vi "Test - Draw Teapot.vi"() -> ()   [LabVIEW 2022 SP3, in "Raster.lvlib"] (continued)
"UV"={"u"=0.0, "v"=0.0}, "Colour"=12517256}, "Vertex 2"={"Position"={"x"=274.62903, "y"=381.50693, "z"=0.99085957}, "UV"={"u"=0.0, "v"=0.0}, "Colour"=12517256}, "Vertex 3"={"Position"={"x"=264.3577, "y"=384.847, "z"=0.9904829}, "UV"={"u"=0.0, "v"=0.0}, "Colour"=12517256}, "Alpha"=0.0, "Alpha Blending Enabled"=FALSE, "Colour"=6654024}, {"Vertex 1"={"Position"={"x"=274.78113, "y"=379.6353, "z"=0.99085855}, "UV"={"u"=0.0, "v"=0.0}, "Colour"=12517256}, "Vertex 2"={"Position"={"x"=274.32074, "y"=376.97778, "z"=0.99086154}, "UV"={"u"=0.0, "v"=0.0}, "Colour"=12517256}, "Vertex 3"={"Position"={"x"=264.01044, "y"=380.14035, "z"=0.99048406}, "UV"={"u"=0.0, "v"=0.0}, "Colour"=12517256}, "Alpha"=0.0, "Alpha Blending Enabled"=FALSE, "Colour"=329219}, {"Vertex 1"={"Position"={"x"=525.67926, "y"=376.97778, "z"=0.99086154}, "UV"={"u"=0.0, "v"=0.0}, "Colour"=12517256}, "Vertex 2"={"Position"={"x"=525.2189, "y"=379.6353, "z"=0.99085855}, "UV"={"u"=0.0, "v"=0.0}, "Colour"=12517256}, "Vertex 3"={"Position"={"x"=535.4709, "y"=382.89456, "z"=0.99048245}, "UV"={"u"=0.0, "v"=0.0}, "Colour"=12517256}, "Alpha"=0.0, "Alpha Blending Enabled"=FALSE, "Colour"=329219}, {"Vertex 1"={"Position"={"x"=525.2189, "y"=379.6353, "z"=0.99085855}, "UV"={"u"=0.0, "v"=0.0}, "Colour"=12517256}, "Vertex 2"={"Position"={"x"=525.371, "y"=381.50693, "z"=0.99085957}, "UV"={"u"=0.0, "v"=0.0}, "Colour"=12517256}, "Vertex 3"={"Position"={"x"=535.6423, "y"=384.847, "z"=0.9904829}, "UV"={"u"=0.0, "v"=0.0}, "Colour"=12517256}, "Alpha"=0.0, "Alpha Blending Enabled"=FALSE, "Colour"=2898719}, {"Vertex 1"={"Position"={"x"=274.62903, "y"=381.50693, "z"=0.99085957}, "UV"={"u"=0.0, "v"=0.0}, "Colour"=12517256}, "Vertex 2"={"Position"={"x"=274.78113, "y"=379.6353, "z"=0.99085855}, "UV"={"u"=0.0, "v"=0.0}, "Colour"=12517256}, "Vertex 3"={"Position"={"x"=264.52908, "y"=382.89456, "z"=0.99048245}, "UV"={"u"=0.0, "v"=0.0}, "Colour"=12517256}, "Alpha"=0.0, "Alpha Blending Enabled"=FALSE, "Colour"=2898719}, {"Vertex 1"={"Position"={"x"=263.60925, "y"=385.99985, "z"=0.99048537}, "UV"={"u"=0.0, "v"=0.0}, "Colour"=12517256}, "Vertex 2"={"Position"={"x"=262.39697, "y"=386.3562, "z"=0.99048924}, "UV"={"u"=0.0, "v"=0.0}, "Colour"=12517256}, "Vertex 3"={"Position"={"x"=272.88913, "y"=382.90955, "z"=0.99087083}, "UV"={"u"=0.0, "v"=0.0}, "Colour"=12517256}, "Alpha"=0.0, "Alpha Blending Enabled"=FALSE, "Colour"=9091427}, {"Vertex 1"={"Position"={"x"=535.98956, "y"=380.14035, "z"=0.99048406}, "UV"={"u"=0.0, "v"=0.0}, "Colour"=12517256}, "Vertex 2"={"Position"={"x"=537.31, "y"=376.584, "z"=0.9904883}, "UV"={"u"=0.0, "v"=0.0}, "Colour"=12517256}, "Vertex 3"={"Position"={"x"=526.851, "y"=373.53363, "z"=0.99086916}, "UV"={"u"=0.0, "v"=0.0}, "Colour"=12517256}, "Alpha"=0.0, "Alpha Blending Enabled"=FALSE, "Colour"=131841}, {"Vertex 1"={"Position"={"x"=537.603, "y"=386.3562, "z"=0.99048924}, "UV"={"u"=0.0, "v"=0.0}, "Colour"=12517256}, "Vertex 2"={"Position"={"x"=536.39075, "y"=385.99985, "z"=0.99048537}, "UV"={"u"=0.0, "v"=0.0}, "Colour"=12517256}, "Vertex 3"={"Position"={"x"=526.03534, "y"=382.5964, "z"=0.9908639}, "UV"={"u"=0.0, "v"=0.0}, "Colour"=12517256}, "Alpha"=0.0, "Alpha Blending Enabled"=FALSE, "Colour"=9091427}, {"Vertex 1"={"Position"={"x"=262.69003, "y"=376.584, "z"=0.9904883}, "UV"={"u"=0.0, "v"=0.0}, "Colour"=12517256}, "Vertex 2"={"Position"={"x"=264.01044, "y"=380.14035, "z"=0.99048406}, "UV"={"u"=0.0, "v"=0.0}, "Colour"=12517256}, "Vertex 3"={"Position"={"x"=274.32074, "y"=376.97778, "z"=0.99086154}, "UV"={"u"=0.0, "v"=0.0}, "Colour"=12517256}, "Alpha"=0.0, "Alpha Blending Enabled"=FALSE, "Colour"=131841}, {"Vertex 1"={"Position"={"x"=264.3577, "y"=384.847, "z"=0.9904829}, "UV"={"u"=0.0, "v"=0.0}, "Colour"=12517256}, "Vertex 2"={"Position"={"x"=263.60925, "y"=385.99985, "z"=0.99048537}, "UV"={"u"=0.0, "v"=0.0}, "Colour"=12517256}, "Vertex 3"={"Position"={"x"=273.96463, "y"=382.5964, "z"=0.9908639}, "UV"={"u"=0.0, "v"=0.0}, "Colour"=12517256}, "Alpha"=0.0, "Alpha Blending Enabled"=FALSE, "Colour"=6654024}, {"Vertex 1"={"Position"={"x"=535.4709, "y"=382.89456, "z"=0.99048245}, "UV"={"u"=0.0, "v"=0.0}, "Colour"=12517256}, "Vertex 2"={"Position"={"x"=535.98956, "y"=380.14035, "z"=0.99048406}, "UV"={"u"=0.0, "v"=0.0}, "Colour"=12517256}, "Vertex 3"={"Position"={"x"=525.67926, "y"=376.97778, "z"=0.99086154}, "UV"={"u"=0.0, "v"=0.0}, "Colour"=12517256}, "Alpha"=0.0, "Alpha Blending Enabled"=FALSE, "Colour"=329219}, {"Vertex 1"={"Position"={"x"=536.39075, "y"=385.99985, "z"=0.99048537}, "UV"={"u"=0.0, "v"=0.0}, "Colour"=12517256}, "Vertex 2"={"Position"={"x"=535.6423, "y"=384.847, "z"=0.9904829}, "UV"={"u"=0.0, "v"=0.0}, "Colour"=12517256}, "Vertex 3"={"Position"={"x"=525.371, "y"=381.50693, "z"=0.99085957}, "UV"={"u"=0.0, "v"=0.0}, "Colour"=12517256}, "Alpha"=0.0, "Alpha Blending Enabled"=FALSE, "Colour"=6654024}, {"Vertex 1"={"Position"={"x"=264.01044, "y"=380.14035, "z"=0.99048406}, "UV"={"u"=0.0, "v"=0.0}, "Colour"=12517256}, "Vertex 2"={"Position"={"x"=264.52908, "y"=382.89456, "z"=0.99048245}, "UV"={"u"=0.0, "v"=0.0}, "Colour"=12517256}, "Vertex 3"={"Position"={"x"=274.78113, "y"=379.6353, "z"=0.99085855}, "UV"={"u"=0.0, "v"=0.0}, "Colour"=12517256}, "Alpha"=0.0, "Alpha Blending Enabled"=FALSE, "Colour"=329219}, {"Vertex 1"={"Position"={"x"=264.52908, "y"=382.89456, "z"=0.99048245}, "UV"={"u"=0.0, "v"=0.0}, "Colour"=12517256}, "Vertex 2"={"Position"={"x"=264.3577, "y"=384.847, "z"=0.9904829}, "UV"={"u"=0.0, "v"=0.0}, "Colour"=12517256}, "Vertex 3"={"Position"={"x"=274.62903, "y"=381.50693, "z"=0.99085957}, "UV"={"u"=0.0, "v"=0.0}, "Colour"=12517256}, "Alpha"=0.0, "Alpha Blending Enabled"=FALSE, "Colour"=2898719}, {"Vertex 1"={"Position"={"x"=535.6423, "y"=384.847, "z"=0.9904829}, "UV"={"u"=0.0, "v"=0.0}, "Colour"=12517256}, "Vertex 2"={"Position"={"x"=535.4709, "y"=382.89456, "z"=0.99048245}, "UV"={"u"=0.0, "v"=0.0}, "Colour"=12517256}, "Vertex 3"={"Position"={"x"=525.2189, "y"=379.6353, "z"=0.99085855}, "UV"={"u"=0.0, "v"=0.0}, "Colour"=12517256}, "Alpha"=0.0, "Alpha Blending Enabled"=FALSE, "Colour"=2898719}, {"Vertex 1"={"Position"={"x"=536.39075, "y"=385.99985, "z"=0.99048537}, "UV"={"u"=0.0, "v"=0.0}, "Colour"=12517256}, "Vertex 2"={"Position"={"x"=537.603, "y"=386.3562, "z"=0.99048924}, "UV"={"u"=0.0, "v"=0.0}, "Colour"=12517256}, "Vertex 3"={"Position"={"x"=545.817, "y"=390.33246, "z"=0.990049}, "UV"={"u"=0.0, "v"=0.0}, "Colour"=12517256}, "Alpha"=0.0, "Alpha Blending Enabled"=FALSE, "Colour"=8696158}, {"Vertex 1"={"Position"={"x"=262.39697, "y"=386.3562, "z"=0.99048924}, "UV"={"u"=0.0, "v"=0.0}, "Colour"=12517256}, "Vertex 2"={"Position"={"x"=263.60925, "y"=385.99985, "z"=0.99048537}, "UV"={"u"=0.0, "v"=0.0}, "Colour"=12517256}, "Vertex 3"={"Position"={"x"=255.52615, "y"=389.92322, "z"=0.990049}, "UV"={"u"=0.0, "v"=0.0}, "Colour"=12517256}, "Alpha"=0.0, "Alpha Blending Enabled"=FALSE, "Colour"=8696158}, {"Vertex 1"={"Position"={"x"=537.31, "y"=376.584, "z"=0.9904883}, "UV"={"u"=0.0, "v"=0.0}, "Colour"=12517256}, "Vertex 2"={"Position"={"x"=535.98956, "y"=380.14035, "z"=0.99048406}, "UV"={"u"=0.0, "v"=0.0}, "Colour"=12517256}, "Vertex 3"={"Position"={"x"=544.02954, "y"=383.7852, "z"=0.990049}, "UV"={"u"=0.0, "v"=0.0}, "Colour"=12517256}, "Alpha"=0.0, "Alpha Blending Enabled"=FALSE, "Colour"=131841}, {"Vertex 1"={"Position"={"x"=264.01044, "y"=380.14035, "z"=0.99048406}, "UV"={"u"=0.0, "v"=0.0}, "Colour"=12517256}, "Vertex 2"={"Position"={"x"=262.69003, "y"=376.584, "z"=0.9904883}, "UV"={"u"=0.0, "v"=0.0}, "Colour"=12517256}, "Vertex 3"={"Position"={"x"=254.50774, "y"=380.10245, "z"=0.990049}, "UV"={"u"=0.0, "v"=0.0}, "Colour"=12517256}, "Alpha"=0.0, "Alpha Blending Enabled"=FALSE, "Colour"=131841}, {"Vertex 1"={"Position"={"x"=535.6423, "y"=384.847, "z"=0.9904829}, "UV"={"u"=0.0, "v"=0.0}, "Colour"=12517256}, "Vertex 2"={"Position"={"x"=536.39075, "y"=385.99985, "z"=0.99048537}, "UV"={"u"=0.0, "v"=0.0}, "Colour"=12517256}, "Vertex 3"={"Position"={"x"=544.4738, "y"=389.92322, "z"=0.990049}, "UV"={"u"=0.0, "v"=0.0}, "Colour"=12517256}, "Alpha"=0.0, "Alpha Blending Enabled"=FALSE, "Colour"=5533756}, {"Vertex 1"={"Position"={"x"=263.60925, "y"=385.99985, "z"=0.99048537}, "UV"={"u"=0.0, "v"=0.0}, "Colour"=12517256}, "Vertex 2"={"Position"={"x"=264.3577, "y"=384.847, "z"=0.9904829}, "UV"={"u"=0.0, "v"=0.0}, "Colour"=12517256}, "Vertex 3"={"Position"={"x"=256.35495, "y"=388.6956, "z"=0.990049}, "UV"={"u"=0.0, "v"=0.0}, "Colour"=12517256}, "Alpha"=0.0, "Alpha Blending Enabled"=FALSE, "Colour"=5533756}, {"Vertex 1"={"Position"={"x"=535.98956, "y"=380.14035, "z"=0.99048406}, "UV"={"u"=0.0, "v"=0.0}, "Colour"=12517256}, "Vertex 2"={"Position"={"x"=535.4709, "y"=382.89456, "z"=0.99048245}, "UV"={"u"=0.0, "v"=0.0}, "Colour"=12517256}, "Vertex 3"={"Position"={"x"=543.4554, "y"=386.64966, "z"=0.990049}, "UV"={"u"=0.0, "v"=0.0}, "Colour"=12517256}, "Alpha"=0.0, "Alpha Blending Enabled"=FALSE, "Colour"=131841}, {"Vertex 1"={"Position"={"x"=264.52908, "y"=382.89456, "z"=0.99048245}, "UV"={"u"=0.0, "v"=0.0}, "Colour"=12517256}, "Vertex 2"={"Position"={"x"=264.01044, "y"=380.14035, "z"=0.99048406}, "UV"={"u"=0.0, "v"=0.0}, "Colour"=12517256}, "Vertex 3"={"Position"={"x"=255.97043, "y"=383.7852, "z"=0.990049}, "UV"={"u"=0.0, "v"=0.0}, "Colour"=12517256}, "Alpha"=0.0, "Alpha Blending Enabled"=FALSE, "Colour"=131841}, {"Vertex 1"={"Position"={"x"=535.4709, "y"=382.89456, "z"=0.99048245}, "UV"={"u"=0.0, "v"=0.0}, "Colour"=12517256}, "Vertex 2"={"Position"={"x"=535.6423, "y"=384.847, "z"=0.9904829}, "UV"={"u"=0.0, "v"=0.0}, "Colour"=12517256}, "Vertex 3"={"Position"={"x"=543.645, "y"=388.6956, "z"=0.990049}, "UV"={"u"=0.0, "v"=0.0}, "Colour"=12517256}, "Alpha"=0.0, "Alpha Blending Enabled"=FALSE, "Colour"=1515280}, {"Vertex 1"={"Position"={"x"=264.3577, "y"=384.847, "z"=0.9904829}, "UV"={"u"=0.0, "v"=0.0}, "Colour"=12517256}, "Vertex 2"={"Position"={"x"=264.52908, "y"=382.89456, "z"=0.99048245}, "UV"={"u"=0.0, "v"=0.0}, "Colour"=12517256}, "Vertex 3"={"Position"={"x"=256.54462, "y"=386.64966, "z"=0.990049}, "UV"={"u"=0.0, "v"=0.0}, "Colour"=12517256}, "Alpha"=0.0, "Alpha Blending Enabled"=FALSE, "Colour"=1515280}, {"Vertex 1"={"Position"={"x"=715.71875, "y"=384.4896, "z"=0.9903194}, "UV"={"u"=0.0, "v"=0.0}, "Colour"=12517256}, "Vertex 2"={"Position"={"x"=715.4581, "y"=384.50897, "z"=0.9903403}, "UV"={"u"=0.0, "v"=0.0}, "Colour"=12517256}, "Vertex 3"={"Position"={"x"=724.84296, "y"=384.92288, "z"=0.990329}, "UV"={"u"=0.0, "v"=0.0}, "Colour"=12517256}, "Alpha"=0.0, "Alpha Blending Enabled"=FALSE, "Colour"=10145646}, {"Vertex 1"={"Position"={"x"=707.5032, "y"=384.25742, "z"=0.9903088}, "UV"={"u"=0.0, "v"=0.0}, "Colour"=12517256}, "Vertex 2"={"Position"={"x"=706.80945, "y"=384.29214, "z"=0.990329}, "UV"={"u"=0.0, "v"=0.0}, "Colour"=12517256}, "Vertex 3"={"Position"={"x"=715.4581, "y"=384.50897, "z"=0.9903403}, "UV"={"u"=0.0, "v"=0.0}, "Colour"=12517256}, "Alpha"=0.0, "Alpha Blending Enabled"=FALSE, "Colour"=10409073}, {"Vertex 1"={"Position"={"x"=715.4581, "y"=384.50897, "z"=0.9903403}, "UV"={"u"=0.0, "v"=0.0}, "Colour"=12517256}, "Vertex 2"={"Position"={"x"=715.71875, "y"=384.4896, "z"=0.9903194}, "UV"={"u"=0.0, "v"=0.0}, "Colour"=12517256}, "Vertex 3"={"Position"={"x"=707.5032, "y"=384.25742, "z"=0.9903088}, "UV"={"u"=0.0, "v"=0.0}, "Colour"=12517256}, "Alpha"=0.0, "Alpha Blending Enabled"=FALSE, "Colour"=10211439}, {"Vertex 1"={"Position"={"x"=724.84296, "y"=384.92288, "z"=0.990329}, "UV"={"u"=0.0, "v"=0.0}, "Colour"=12517256}, "Vertex 2"={"Position"={"x"=724.6177, "y"=384.9046, "z"=0.9903088}, "UV"={"u"=0.0, "v"=0.0}, "Colour"=12517256}, "Vertex 3"={"Position"={"x"=715.71875, "y"=384.4896, "z"=0.9903194}, "UV"={"u"=0.0, "v"=0.0}, "Colour"=12517256}, "Alpha"=0.0, "Alpha Blending Enabled"=FALSE, "Colour"=10013805}, {"Vertex 1"={"Position"={"x"=724.6177, "y"=384.9046, "z"=0.9903088}, "UV"={"u"=0.0, "v"=0.0}, "Colour"=12517256}, "Vertex 2"={"Position"={"x"=724.84296, "y"=384.92288, "z"=0.990329}, "UV"={"u"=0.0, "v"=0.0}, "Colour"=12517256}, "Vertex 3"={"Position"={"x"=734.2983, "y"=385.51193, "z"=0.9902948}, "UV"={"u"=0.0, "v"=0.0}, "Colour"=12517256}, "Alpha"=0.0, "Alpha Blending Enabled"=FALSE, "Colour"=9881963}, {"Vertex 1"={"Position"={"x"=714.87616, "y"=383.89682, "z"=0.9903}, "UV"={"u"=0.0, "v"=0.0}, "Colour"=12517256}, "Vertex 2"={"Position"={"x"=715.71875, "y"=384.4896, "z"=0.9903194}, "UV"={"u"=0.0, "v"=0.0}, "Colour"=12517256}, "Vertex 3"={"Position"={"x"=724.6177, "y"=384.9046, "z"=0.9903088}, "UV"={"u"=0.0, "v"=0.0}, "Colour"=12517256}, "Alpha"=0.0, "Alpha Blending Enabled"=FALSE, "Colour"=12187780}, {"Vertex 1"={"Position"={"x"=707.1928, "y"=383.67975, "z"=0.99029016}, "UV"={"u"=0.0, "v"=0.0}, "Colour"=12517256}, "Vertex 2"={"Position"={"x"=707.5032, "y"=384.25742, "z"=0.9903088}, "UV"={"u"=0.0, "v"=0.0}, "Colour"=12517256}, "Vertex 3"={"Position"={"x"=715.71875, "y"=384.4896, "z"=0.9903194}, "UV"={"u"=0.0, "v"=0.0}, "Colour"=12517256}, "Alpha"=0.0, "Alpha Blending Enabled"=FALSE, "Colour"=12385671}, {"Vertex 1"={"Position"={"x"=706.80945, "y"=384.29214, "z"=0.990329}, "UV"={"u"=0.0, "v"=0.0}, "Colour"=12517256}, "Vertex 2"={"Position"={"x"=707.5032, "y"=384.25742, "z"=0.9903088}, "UV"={"u"=0.0, "v"=0.0}, "Colour"=12517256}, "Vertex 3"={"Position"={"x"=700.6159, "y"=384.23364, "z"=0.99027705}, "UV"={"u"=0.0, "v"=0.0}, "Colour"=12517256}, "Alpha"=0.0, "Alpha Blending Enabled"=FALSE, "Colour"=10343281}, {"Vertex 1"={"Position"={"x"=715.71875, "y"=384.4896, "z"=0.9903194}, "UV"={"u"=0.0, "v"=0.0}, "Colour"=12517256}, "Vertex 2"={"Position"={"x"=714.87616, "y"=383.89682, "z"=0.9903}, "UV"={"u"=0.0, "v"=0.0}, "Colour"=12517256}, "Vertex 3"={"Position"={"x"=707.1928, "y"=383.67975, "z"=0.99029016}, "UV"={"u"=0.0, "v"=0.0}, "Colour"=12517256}, "Alpha"=0.0, "Alpha Blending Enabled"=FALSE, "Colour"=12385415}, {"Vertex 1"={"Position"={"x"=700.6159, "y"=384.23364, "z"=0.99027705}, "UV"={"u"=0.0, "v"=0.0}, "Colour"=12517256}, "Vertex 2"={"Position"={"x"=699.572, "y"=384.29733, "z"=0.9902948}, "UV"={"u"=0.0, "v"=0.0}, "Colour"=12517256}, "Vertex 3"={"Position"={"x"=706.80945, "y"=384.29214, "z"=0.990329}, "UV"={"u"=0.0, "v"=0.0}, "Colour"=12517256}, "Alpha"=0.0, "Alpha Blending Enabled"=FALSE, "Colour"=10540915}, {"Vertex 1"={"Position"={"x"=724.6177, "y"=384.9046, "z"=0.9903088}, "UV"={"u"=0.0, "v"=0.0}, "Colour"=12517256}, "Vertex 2"={"Position"={"x"=723.1924, "y"=384.28253, "z"=0.99029016}, "UV"={"u"=0.0, "v"=0.0}, "Colour"=12517256}, "Vertex 3"={"Position"={"x"=714.87616, "y"=383.89682, "z"=0.9903}, "UV"={"u"=0.0, "v"=0.0}, "Colour"=12517256}, "Alpha"=0.0, "Alpha Blending Enabled"=FALSE, "Colour"=12187780}, {"Vertex 1"={"Position"={"x"=734.2983, "y"=385.51193, "z"=0.9902948}, "UV"={"u"=0.0, "v"=0.0}, "Colour"=12517256}, "Vertex 2"={"Position"={"x"=733.564, "y"=385.4795, "z"=0.99027705}, "UV"={"u"=0.0, "v"=0.0}, "Colour"=12517256}, "Vertex 3"={"Position"={"x"=724.6177, "y"=384.9046, "z"=0.9903088}, "UV"={"u"=0.0, "v"=0.0}, "Colour"=12517256}, "Alpha"=0.0, "Alpha Blending Enabled"=FALSE, "Colour"=9750378}, {"Vertex 1"={"Position"={"x"=723.1924, "y"=384.28253, "z"=0.99029016}, "UV"={"u"=0.0, "v"=0.0}, "Colour"=12517256}, "Vertex 2"={"Position"={"x"=724.6177, "y"=384.9046, "z"=0.9903088}, "UV"={"u"=0.0, "v"=0.0}, "Colour"=12517256}, "Vertex 3"={"Position"={"x"=733.564, "y"=385.4795, "z"=0.99027705}, "UV"={"u"=0.0, "v"=0.0}, "Colour"=12517256}, "Alpha"=0.0, "Alpha Blending Enabled"=FALSE, "Colour"=11726976}, {"Vertex 1"={"Position"={"x"=712.84686, "y"=382.6958, "z"=0.99028397}, "UV"={"u"=0.0, "v"=0.0}, "Colour"=12517256}, "Vertex 2"={"Position"={"x"=714.87616, "y"=383.89682, "z"=0.9903}, "UV"={"u"=0.0, "v"=0.0}, "Colour"=12517256}, "Vertex 3"={"Position"={"x"=723.1924, "y"=384.28253, "z"=0.99029016}, "UV"={"u"=0.0, "v"=0.0}, "Colour"=12517256}, "Alpha"=0.0, "Alpha Blending Enabled"=FALSE, "Colour"=12451207}, {"Vertex 1"={"Position"={"x"=705.7688, "y"=382.53003, "z"=0.9902748}, "UV"={"u"=0.0, "v"=0.0}, "Colour"=12517256}, "Vertex 2"={"Position"={"x"=707.1928, "y"=383.67975, "z"=0.99029016}, "UV"={"u"=0.0, "v"=0.0}, "Colour"=12517256}, "Vertex 3"={"Position"={"x"=714.87616, "y"=383.89682, "z"=0.9903}, "UV"={"u"=0.0, "v"=0.0}, "Colour"=12517256}, "Alpha"=0.0, "Alpha Blending Enabled"=FALSE, "Colour"=12056195}, {"Vertex 1"={"Position"={"x"=707.5032, "y"=384.25742, "z"=0.9903088}, "UV"={"u"=0.0, "v"=0.0}, "Colour"=12517256}, "Vertex 2"={"Position"={"x"=707.1928, "y"=383.67975, "z"=0.99029016}, "UV"={"u"=0.0, "v"=0.0}, "Colour"=12517256}, "Vertex 3"={"Position"={"x"=700.7482, "y"=383.6549, "z"=0.99026066}, "UV"={"u"=0.0, "v"=0.0}, "Colour"=12517256}, "Alpha"=0.0, "Alpha Blending Enabled"=FALSE, "Colour"=12385671}, {"Vertex 1"={"Position"={"x"=714.87616, "y"=383.89682, "z"=0.9903}, "UV"={"u"=0.0, "v"=0.0}, "Colour"=12517256}, "Vertex 2"={"Position"={"x"=712.84686, "y"=382.6958, "z"=0.99028397}, "UV"={"u"=0.0, "v"=0.0}, "Colour"=12517256}, "Vertex 3"={"Position"={"x"=705.7688, "y"=382.53003, "z"=0.9902748}, "UV"={"u"=0.0, "v"=0.0}, "Colour"=12517256}, "Alpha"=0.0, "Alpha Blending Enabled"=FALSE, "Colour"=11990146}, {"Vertex 1"={"Position"={"x"=723.1924, "y"=384.28253, "z"=0.99029016}, "UV"={"u"=0.0, "v"=0.0}, "Colour"=12517256}, "Vertex 2"={"Position"={"x"=720.51355, "y"=383.01724, "z"=0.9902748}, "UV"={"u"=0.0, "v"=0.0}, "Colour"=12517256}, "Vertex 3"={"Position"={"x"=712.84686, "y"=382.6958, "z"=0.99028397}, "UV"={"u"=0.0, "v"=0.0}, "Colour"=12517256}, "Alpha"=0.0, "Alpha Blending Enabled"=FALSE, "Colour"=12385671}, {"Vertex 1"={"Position"={"x"=700.7482, "y"=383.6549, "z"=0.99026066}, "UV"={"u"=0.0, "v"=0.0}, "Colour"=12517256}, "Vertex 2"={"Position"={"x"=700.6159, "y"=384.23364, "z"=0.99027705}, "UV"={"u"=0.0, "v"=0.0}, "Colour"=12517256}, "Vertex 3"={"Position"={"x"=707.5032, "y"=384.25742, "z"=0.9903088}, "UV"={"u"=0.0, "v"=0.0}, "Colour"=12517256}, "Alpha"=0.0, "Alpha Blending Enabled"=FALSE, "Colour"=12385671}, {"Vertex 1"={"Position"={"x"=709.5495, "y"=380.85352, "z"=0.9902731}, "UV"={"u"=0.0, "v"=0.0}, "Colour"=12517256}, "Vertex 2"={"Position"={"x"=712.84686, "y"=382.6958, "z"=0.99028397}, "UV"={"u"=0.0, "v"=0.0}, "Colour"=12517256}, "Vertex 3"={"Position"={"x"=720.51355, "y"=383.01724, "z"=0.9902748}, "UV"={"u"=0.0, "v"=0.0}, "Colour"=12517256}, "Alpha"=0.0, "Alpha Blending Enabled"=FALSE, "Colour"=11660927}, {"Vertex 1"={"Position"={"x"=733.564, "y"=385.4795, "z"=0.99027705}, "UV"={"u"=0.0, "v"=0.0}, "Colour"=12517256}, "Vertex 2"={"Position"={"x"=731.54297, "y"=384.81516, "z"=0.99026066}, "UV"={"u"=0.0, "v"=0.0}, "Colour"=12517256}, "Vertex 3"={"Position"={"x"=723.1924, "y"=384.28253, "z"=0.99029016}, "UV"={"u"=0.0, "v"=0.0}, "Colour"=12517256}, "Alpha"=0.0, "Alpha Blending Enabled"=FALSE, "Colour"=11792512}, {"Vertex 1"={"Position"={"x"=720.51355, "y"=383.01724, "z"=0.9902748}, "UV"={"u"=0.0, "v"=0.0}, "Colour"=12517256}, "Vertex 2"={"Position"={"x"=723.1924, "y"=384.28253, "z"=0.99029016}, "UV"={"u"=0.0, "v"=0.0}, "Colour"=12517256}, "Vertex 3"={"Position"={"x"=731.54297, "y"=384.81516, "z"=0.99026066}, "UV"={"u"=0.0, "v"=0.0}, "Colour"=12517256}, "Alpha"=0.0, "Alpha Blending Enabled"=FALSE, "Colour"=12319622}, {"Vertex 1"={"Position"={"x"=703.12384, "y"=380.78134, "z"=0.9902643}, "UV"={"u"=0.0, "v"=0.0}, "Colour"=12517256}, "Vertex 2"={"Position"={"x"=705.7688, "y"=382.53003, "z"=0.9902748}, "UV"={"u"=0.0, "v"=0.0}, "Colour"=12517256}, "Vertex 3"={"Position"={"x"=712.84686, "y"=382.6958, "z"=0.99028397}, "UV"={"u"=0.0, "v"=0.0}, "Colour"=12517256}, "Alpha"=0.0, "Alpha Blending Enabled"=FALSE, "Colour"=10409329}, {"Vertex 1"={"Position"={"x"=712.84686, "y"=382.6958, "z"=0.99028397}, "UV"={"u"=0.0, "v"=0.0}, "Colour"=12517256}, "Vertex 2"={"Position"={"x"=709.5495, "y"=380.85352, "z"=0.9902731}, "UV"={"u"=0.0, "v"=0.0}, "Colour"=12517256}, "Vertex 3"={"Position"={"x"=703.12384, "y"=380.78134, "z"=0.9902643}, "UV"={"u"=0.0, "v"=0.0}, "Colour"=12517256}, "Alpha"=0.0, "Alpha Blending Enabled"=FALSE, "Colour"=10211439}, {"Vertex 1"={"Position"={"x"=720.51355, "y"=383.01724, "z"=0.9902748}, "UV"={"u"=0.0, "v"=0.0}, "Colour"=12517256}, "Vertex 2"={"Position"={"x"=716.53064, "y"=381.07083, "z"=0.9902643}, "UV"={"u"=0.0, "v"=0.0}, "Colour"=12517256}, "Vertex 3"={"Position"={"x"=709.5495, "y"=380.85352, "z"=0.9902731}, "UV"={"u"=0.0, "v"=0.0}, "Colour"=12517256}, "Alpha"=0.0, "Alpha Blending Enabled"=FALSE, "Colour"=11660670}, {"Vertex 1"={"Position"={"x"=707.1928, "y"=383.67975, "z"=0.99029016}, "UV"={"u"=0.0, "v"=0.0}, "Colour"=12517256}, "Vertex 2"={"Position"={"x"=705.7688, "y"=382.53003, "z"=0.9902748}, "UV"={"u"=0.0, "v"=0.0}, "Colour"=12517256}, "Vertex 3"={"Position"={"x"=699.84033, "y"=382.53918, "z"=0.99024713}, "UV"={"u"=0.0, "v"=0.0}, "Colour"=12517256}, "Alpha"=0.0, "Alpha Blending Enabled"=FALSE, "Colour"=11001975}, {"Vertex 1"={"Position"={"x"=733.564, "y"=385.4795, "z"=0.99027705}, "UV"={"u"=0.0, "v"=0.0}, "Colour"=12517256}, "Vertex 2"={"Position"={"x"=734.2983, "y"=385.51193, "z"=0.9902948}, "UV"={"u"=0.0, "v"=0.0}, "Colour"=12517256}, "Vertex 3"={"Position"={"x"=743.1542, "y"=386.25623, "z"=0.9902374}, "UV"={"u"=0.0, "v"=0.0}, "Colour"=12517256}, "Alpha"=0.0, "Alpha Blending Enabled"=FALSE, "Colour"=9618280}, {"Vertex 1"={"Position"={"x"=704.9087, "y"=378.3398, "z"=0.99026906}, "UV"={"u"=0.0, "v"=0.0}, "Colour"=12517256}, "Vertex 2"={"Position"={"x"=709.5495, "y"=380.85352, "z"=0.9902731}, "UV"={"u"=0.0, "v"=0.0}, "Colour"=12517256}, "Vertex 3"={"Position"={"x"=716.53064, "y"=381.07083, "z"=0.9902643}, "UV"={"u"=0.0, "v"=0.0}, "Colour"=12517256}, "Alpha"=0.0, "Alpha Blending Enabled"=FALSE, "Colour"=10540914}, {"Vertex 1"={"Position"={"x"=709.5495, "y"=380.85352, "z"=0.9902731}, "UV"={"u"=0.0, "v"=0.0}, "Colour"=12517256}, "Vertex 2"={"Position"={"x"=704.9087, "y"=378.3398, "z"=0.99026906}, "UV"={"u"=0.0, "v"=0.0}, "Colour"=12517256}, "Vertex 3"={"Position"={"x"=699.15515, "y"=378.40884, "z"=0.9902605}, "UV"={"u"=0.0, "v"=0.0}, "Colour"=12517256}, "Alpha"=0.0, "Alpha Blending Enabled"=FALSE, "Colour"=8300890}, {"Vertex 1"={"Position"={"x"=699.15515, "y"=378.40884, "z"=0.9902605}, "UV"={"u"=0.0, "v"=0.0}, "Colour"=12517256}, "Vertex 2"={"Position"={"x"=703.12384, "y"=380.78134, "z"=0.9902643}, "UV"={"u"=0.0, "v"=0.0}, "Colour"=12517256}, "Vertex 3"={"Position"={"x"=709.5495, "y"=380.85352, "z"=0.9902731}, "UV"={"u"=0.0, "v"=0.0}, "Colour"=12517256}, "Alpha"=0.0, "Alpha Blending Enabled"=FALSE, "Colour"=8498781}, {"Vertex 1"={"Position"={"x"=699.84033, "y"=382.53918, "z"=0.99024713}, "UV"={"u"=0.0, "v"=0.0}, "Colour"=12517256}, "Vertex 2"={"Position"={"x"=700.7482, "y"=383.6549, "z"=0.99026066}, "UV"={"u"=0.0, "v"=0.0}, "Colour"=12517256}, "Vertex 3"={"Position"={"x"=707.1928, "y"=383.67975, "z"=0.99029016}, "UV"={"u"=0.0, "v"=0.0}, "Colour"=12517256}, "Alpha"=0.0, "Alpha Blending Enabled"=FALSE, "Colour"=11199609}, {"Vertex 1"={"Position"={"x"=699.572, "y"=384.29733, "z"=0.9902948}, "UV"={"u"=0.0, "v"=0.0}, "Colour"=12517256}, "Vertex 2"={"Position"={"x"=700.6159, "y"=384.23364, "z"=0.99027705}, "UV"={"u"=0.0, "v"=0.0}, "Colour"=12517256}, "Vertex 3"={"Position"={"x"=695.72473, "y"=384.44632, "z"=0.9902237}, "UV"={"u"=0.0, "v"=0.0}, "Colour"=12517256}, "Alpha"=0.0, "Alpha Blending Enabled"=FALSE, "Colour"=10409073}, {"Vertex 1"={"Position"={"x"=716.53064, "y"=381.07083, "z"=0.9902643}, "UV"={"u"=0.0, "v"=0.0}, "Colour"=12517256}, "Vertex 2"={"Position"={"x"=711.1995, "y"=378.40884, "z"=0.9902605}, "UV"={"u"=0.0, "v"=0.0}, "Colour"=12517256}, "Vertex 3"={"Position"={"x"=704.9087, "y"=378.3398, "z"=0.99026906}, "UV"={"u"=0.0, "v"=0.0}, "Colour"=12517256}, "Alpha"=0.0, "Alpha Blending Enabled"=FALSE, "Colour"=10606707}, {"Vertex 1"={"Position"={"x"=716.53064, "y"=381.07083, "z"=0.9902643}, "UV"={"u"=0.0, "v"=0.0}, "Colour"=12517256}, "Vertex 2"={"Position"={"x"=720.51355, "y"=383.01724, "z"=0.9902748}, "UV"={"u"=0.0, "v"=0.0}, "Colour"=12517256}, "Vertex 3"={"Position"={"x"=728.21436, "y"=383.47656, "z"=0.99024713}, "UV"={"u"=0.0, "v"=0.0}, "Colour"=12517256}, "Alpha"=0.0, "Alpha Blending Enabled"=FALSE, "Colour"=12188037}, {"Vertex 1"={"Position"={"x"=731.54297, "y"=384.81516, "z"=0.99026066}, "UV"={"u"=0.0, "v"=0.0}, "Colour"=12517256}, "Vertex 2"={"Position"={"x"=728.21436, "y"=383.47656, "z"=0.99024713}, "UV"={"u"=0.0, "v"=0.0}, "Colour"=12517256}, "Vertex 3"={"Position"={"x"=720.51355, "y"=383.01724, "z"=0.9902748}, "UV"={"u"=0.0, "v"=0.0}, "Colour"=12517256}, "Alpha"=0.0, "Alpha Blending Enabled"=FALSE, "Colour"=12319622}, {"Vertex 1"={"Position"={"x"=705.7688, "y"=382.53003, "z"=0.9902748}, "UV"={"u"=0.0, "v"=0.0}, "Colour"=12517256}, "Vertex 2"={"Position"={"x"=703.12384, "y"=380.78134, "z"=0.9902643}, "UV"={"u"=0.0, "v"=0.0}, "Colour"=12517256}, "Vertex 3"={"Position"={"x"=697.7654, "y"=380.866, "z"=0.99023795}, "UV"={"u"=0.0, "v"=0.0}, "Colour"=12517256}, "Alpha"=0.0, "Alpha Blending Enabled"=FALSE, "Colour"=8037463}, {"Vertex 1"={"Position"={"x"=711.1995, "y"=378.40884, "z"=0.9902605}, "UV"={"u"=0.0, "v"=0.0}, "Colour"=12517256}, "Vertex 2"={"Position"={"x"=716.53064, "y"=381.07083, "z"=0.9902643}, "UV"={"u"=0.0, "v"=0.0}, "Colour"=12517256}, "Vertex 3"={"Position"={"x"=723.5613, "y"=381.423, "z"=0.99023795}, "UV"={"u"=0.0, "v"=0.0}, "Colour"=12517256}, "Alpha"=0.0, "Alpha Blending Enabled"=FALSE, "Colour"=11792512}, {"Vertex 1"={"Position"={"x"=731.54297, "y"=384.81516, "z"=0.99026066}, "UV"={"u"=0.0, "v"=0.0}, "Colour"=12517256}, "Vertex 2"={"Position"={"x"=733.564, "y"=385.4795, "z"=0.99027705}, "UV"={"u"=0.0, "v"=0.0}, "Colour"=12517256}, "Vertex 3"={"Position"={"x"=741.91724, "y"=386.1932, "z"=0.9902237}, "UV"={"u"=0.0, "v"=0.0}, "Colour"=12517256}, "Alpha"=0.0, "Alpha Blending Enabled"=FALSE, "Colour"=11133817}, {"Vertex 1"={"Position"={"x"=697.7654, "y"=380.866, "z"=0.99023795}, "UV"={"u"=0.0, "v"=0.0}, "Colour"=12517256}, "Vertex 2"={"Position"={"x"=699.84033, "y"=382.53918, "z"=0.99024713}, "UV"={"u"=0.0, "v"=0.0}, "Colour"=12517256}, "Vertex 3"={"Position"={"x"=705.7688, "y"=382.53003, "z"=0.9902748}, "UV"={"u"=0.0, "v"=0.0}, "Colour"=12517256}, "Alpha"=0.0, "Alpha Blending Enabled"=FALSE, "Colour"=8564317}, {"Vertex 1"={"Position"={"x"=703.12384, "y"=380.78134, "z"=0.9902643}, "UV"={"u"=0.0, "v"=0.0}, "Colour"=12517256}, "Vertex 2"={"Position"={"x"=699.15515, "y"=378.40884, "z"=0.9902605}, "UV"={"u"=0.0, "v"=0.0}, "Colour"=12517256}, "Vertex 3"={"Position"={"x"=694.39935, "y"=378.6166, "z"=0.99023455}, "UV"={"u"=0.0, "v"=0.0}, "Colour"=12517256}, "Alpha"=0.0, "Alpha Blending Enabled"=FALSE, "Colour"=5402171}, {"Vertex 1"={"Position"={"x"=695.72473, "y"=384.44632, "z"=0.9902237}, "UV"={"u"=0.0, "v"=0.0}, "Colour"=12517256}, "Vertex 2"={"Position"={"x"=694.4478, "y"=384.55273, "z"=0.9902374}, "UV"={"u"=0.0, "v"=0.0}, "Colour"=12517256}, "Vertex 3"={"Position"={"x"=699.572, "y"=384.29733, "z"=0.9902948}, "UV"={"u"=0.0, "v"=0.0}, "Colour"=12517256}, "Alpha"=0.0, "Alpha Blending Enabled"=FALSE, "Colour"=10606707}, {"Vertex 1"={"Position"={"x"=728.21436, "y"=383.47656, "z"=0.99024713}, "UV"={"u"=0.0, "v"=0.0}, "Colour"=12517256}, "Vertex 2"={"Position"={"x"=723.5613, "y"=381.423, "z"=0.99023795}, "UV"={"u"=0.0, "v"=0.0}, "Colour"=12517256}, "Vertex 3"={"Position"={"x"=716.53064, "y"=381.07083, "z"=0.9902643}, "UV"={"u"=0.0, "v"=0.0}, "Colour"=12517256}, "Alpha"=0.0, "Alpha Blending Enabled"=FALSE, "Colour"=12188037}, {"Vertex 1"={"Position"={"x"=700.6159, "y"=384.23364, "z"=0.99027705}, "UV"={"u"=0.0, "v"=0.0}, "Colour"=12517256}, "Vertex 2"={"Position"={"x"=700.7482, "y"=383.6549, "z"=0.99026066}, "UV"={"u"=0.0, "v"=0.0}, "Colour"=12517256}, "Vertex 3"={"Position"={"x"=696.16833, "y"=383.84857, "z"=0.9902111}, "UV"={"u"=0.0, "v"=0.0}, "Colour"=12517256}, "Alpha"=0.0, "Alpha Blending Enabled"=FALSE, "Colour"=12056195}, {"Vertex 1"={"Position"={"x"=743.1542, "y"=386.25623, "z"=0.9902374}, "UV"={"u"=0.0, "v"=0.0}, "Colour"=12517256}, "Vertex 2"={"Position"={"x"=741.91724, "y"=386.1932, "z"=0.9902237}, "UV"={"u"=0.0, "v"=0.0}, "Colour"=12517256}, "Vertex 3"={"Position"={"x"=733.564, "y"=385.4795, "z"=0.99027705}, "UV"={"u"=0.0, "v"=0.0}, "Colour"=12517256}, "Alpha"=0.0, "Alpha Blending Enabled"=FALSE, "Colour"=9486951}, {"Vertex 1"={"Position"={"x"=694.39935, "y"=378.6166, "z"=0.99023455}, "UV"={"u"=0.0, "v"=0.0}, "Colour"=12517256}, "Vertex 2"={"Position"={"x"=697.7654, "y"=380.866, "z"=0.99023795}, "UV"={"u"=0.0, "v"=0.0}, "Colour"=12517256}, "Vertex 3"={"Position"={"x"=703.12384, "y"=380.78134, "z"=0.9902643}, "UV"={"u"=0.0, "v"=0.0}, "Colour"=12517256}, "Alpha"=0.0, "Alpha Blending Enabled"=FALSE, "Colour"=6060865}, {"Vertex 1"={"Position"={"x"=723.5613, "y"=381.423, "z"=0.99023795}, "UV"={"u"=0.0, "v"=0.0}, "Colour"=12517256}, "Vertex 2"={"Position"={"x"=717.57275, "y"=378.6166, "z"=0.99023455}, "UV"={"u"=0.0, "v"=0.0}, "Colour"=12517256}, "Vertex 3"={"Position"={"x"=711.1995, "y"=378.40884, "z"=0.9902605}, "UV"={"u"=0.0, "v"=0.0}, "Colour"=12517256}, "Alpha"=0.0, "Alpha Blending Enabled"=FALSE, "Colour"=11858561}, {"Vertex 1"={"Position"={"x"=728.21436, "y"=383.47656, "z"=0.99024713}, "UV"={"u"=0.0, "v"=0.0}, "Colour"=12517256}, "Vertex 2"={"Position"={"x"=731.54297, "y"=384.81516, "z"=0.99026066}, "UV"={"u"=0.0, "v"=0.0}, "Colour"=12517256}, "Vertex 3"={"Position"={"x"=739.32513, "y"=385.47467, "z"=0.9902111}, "UV"={"u"=0.0, "v"=0.0}, "Colour"=12517256}, "Alpha"=0.0, "Alpha Blending Enabled"=FALSE, "Colour"=11726463}, {"Vertex 1"={"Position"={"x"=696.16833, "y"=383.84857, "z"=0.9902111}, "UV"={"u"=0.0, "v"=0.0}, "Colour"=12517256}, "Vertex 2"={"Position"={"x"=695.72473, "y"=384.44632, "z"=0.9902237}, "UV"={"u"=0.0, "v"=0.0}, "Colour"=12517256}, "Vertex 3"={"Position"={"x"=700.6159, "y"=384.23364, "z"=0.99027705}, "UV"={"u"=0.0, "v"=0.0}, "Colour"=12517256}, "Alpha"=0.0, "Alpha Blending Enabled"=FALSE, "Colour"=12055939}, {"Vertex 1"={"Position"={"x"=700.7482, "y"=383.6549, "z"=0.99026066}, "UV"={"u"=0.0, "v"=0.0}, "Colour"=12517256}, "Vertex 2"={"Position"={"x"=699.84033, "y"=382.53918, "z"=0.99024713}, "UV"={"u"=0.0, "v"=0.0}, "Colour"=12517256}, "Vertex 3"={"Position"={"x"=695.63995, "y"=382.74472, "z"=0.9902007}, "UV"={"u"=0.0, "v"=0.0}, "Colour"=12517256}, "Alpha"=0.0, "Alpha Blending Enabled"=FALSE, "Colour"=9025634}, {"Vertex 1"={"Position"={"x"=741.91724, "y"=386.1932, "z"=0.9902237}, "UV"={"u"=0.0, "v"=0.0}, "Colour"=12517256}, "Vertex 2"={"Position"={"x"=739.32513, "y"=385.47467, "z"=0.9902111}, "UV"={"u"=0.0, "v"=0.0}, "Colour"=12517256}, "Vertex 3"={"Position"={"x"=731.54297, "y"=384.81516, "z"=0.99026066}, "UV"={"u"=0.0, "v"=0.0}, "Colour"=12517256}, "Alpha"=0.0, "Alpha Blending Enabled"=FALSE, "Colour"=11133817}, {"Vertex 1"={"Position"={"x"=723.5613, "y"=381.423, "z"=0.99023795}, "UV"={"u"=0.0, "v"=0.0}, "Colour"=12517256}, "Vertex 2"={"Position"={"x"=728.21436, "y"=383.47656, "z"=0.99024713}, "UV"={"u"=0.0, "v"=0.0}, "Colour"=12517256}, "Vertex 3"={"Position"={"x"=735.3911, "y"=384.05777, "z"=0.9902007}, "UV"={"u"=0.0, "v"=0.0}, "Colour"=12517256}, "Alpha"=0.0, "Alpha Blending Enabled"=FALSE, "Colour"=11924097}, {"Vertex 1"={"Position"={"x"=699.84033, "y"=382.53918, "z"=0.99024713}, "UV"={"u"=0.0, "v"=0.0}, "Colour"=12517256}, "Vertex 2"={"Position"={"x"=697.7654, "y"=380.866, "z"=0.99023795}, "UV"={"u"=0.0, "v"=0.0}, "Colour"=12517256}, "Vertex 3"={"Position"={"x"=694.001, "y"=381.1209, "z"=0.9901936}, "UV"={"u"=0.0, "v"=0.0}, "Colour"=12517256}, "Alpha"=0.0, "Alpha Blending Enabled"=FALSE, "Colour"=4941110}, {"Vertex 1"={"Position"={"x"=695.63995, "y"=382.74472, "z"=0.9902007}, "UV"={"u"=0.0, "v"=0.0}, "Colour"=12517256}, "Vertex 2"={"Position"={"x"=696.16833, "y"=383.84857, "z"=0.9902111}, "UV"={"u"=0.0, "v"=0.0}, "Colour"=12517256}, "Vertex 3"={"Position"={"x"=700.7482, "y"=383.6549, "z"=0.99026066}, "UV"={"u"=0.0, "v"=0.0}, "Colour"=12517256}, "Alpha"=0.0, "Alpha Blending Enabled"=FALSE, "Colour"=9355110}, {"Vertex 1"={"Position"={"x"=717.57275, "y"=378.6166, "z"=0.99023455}, "UV"={"u"=0.0, "v"=0.0}, "Colour"=12517256}, "Vertex 2"={"Position"={"x"=723.5613, "y"=381.423, "z"=0.99023795}, "UV"={"u"=0.0, "v"=0.0}, "Colour"=12517256}, "Vertex 3"={"Position"={"x"=730.1326, "y"=381.90115, "z"=0.9901936}, "UV"={"u"=0.0, "v"=0.0}, "Colour"=12517256}, "Alpha"=0.0, "Alpha Blending Enabled"=FALSE, "Colour"=11924097}, {"Vertex 1"={"Position"={"x"=697.7654, "y"=380.866, "z"=0.99023795}, "UV"={"u"=0.0, "v"=0.0}, "Colour"=12517256}, "Vertex 2"={"Position"={"x"=694.39935, "y"=378.6166, "z"=0.99023455}, "UV"={"u"=0.0, "v"=0.0}, "Colour"=12517256}, "Vertex 3"={"Position"={"x"=691.1157, "y"=378.9654, "z"=0.990191}, "UV"={"u"=0.0, "v"=0.0}, "Colour"=12517256}, "Alpha"=0.0, "Alpha Blending Enabled"=FALSE, "Colour"=2108183}, {"Vertex 1"={"Position"={"x"=739.32513, "y"=385.47467, "z"=0.9902111}, "UV"={"u"=0.0, "v"=0.0}, "Colour"=12517256}, "Vertex 2"={"Position"={"x"=735.3911, "y"=384.05777, "z"=0.9902007}, "UV"={"u"=0.0, "v"=0.0}, "Colour"=12517256}, "Vertex 3"={"Position"={"x"=728.21436, "y"=383.47656, "z"=0.99024713}, "UV"={"u"=0.0, "v"=0.0}, "Colour"=12517256}, "Alpha"=0.0, "Alpha Blending Enabled"=FALSE, "Colour"=11726719}, {"Vertex 1"={"Position"={"x"=694.001, "y"=381.1209, "z"=0.9901936}, "UV"={"u"=0.0, "v"=0.0}, "Colour"=12517256}, "Vertex 2"={"Position"={"x"=695.63995, "y"=382.74472, "z"=0.9902007}, "UV"={"u"=0.0, "v"=0.0}, "Colour"=12517256}, "Vertex 3"={"Position"={"x"=699.84033, "y"=382.53918, "z"=0.99024713}, "UV"={"u"=0.0, "v"=0.0}, "Colour"=12517256}, "Alpha"=0.0, "Alpha Blending Enabled"=FALSE, "Colour"=5731646}, {"Vertex 1"={"Position"={"x"=735.3911, "y"=384.05777, "z"=0.9902007}, "UV"={"u"=0.0, "v"=0.0}, "Colour"=12517256}, "Vertex 2"={"Position"={"x"=730.1326, "y"=381.90115, "z"=0.9901936}, "UV"={"u"=0.0, "v"=0.0}, "Colour"=12517256}, "Vertex 3"={"Position"={"x"=723.5613, "y"=381.423, "z"=0.99023795}, "UV"={"u"=0.0, "v"=0.0}, "Colour"=12517256}, "Alpha"=0.0, 
